vi "Model - Init.vi"(8 "error in (no error)":errorcluster) -> (0 "error out":errorcluster, 3 "View Model":T1)   [LabVIEW 2017]
doc: "Initializes View model's user events and DVRs"
uses:
  Controls/View Model.ctl
  Configuration/Controls/Config Model.ctl
  Configuration/Controls/Config Data.ctl
  Error Handler/Controls/Error Model.ctl
  Error Handler/Controls/Error Data.ctl
  Error Handler/Controls/Error Type.ctl
  Controls/Shared Model.ctl
  Elevator Controller/Controls/Elevator Model.ctl
  Elevator Controller/Controls/Elevator Location.ctl
  Elevator Controller/Controls/Elevator CMD Data.ctl
  Elevator Controller/Controls/Elevator Commands.ctl
  Elevator Controller/Controls/Elevator Overhead.ctl
  Elevator Controller/Controls/Elevator States.ctl
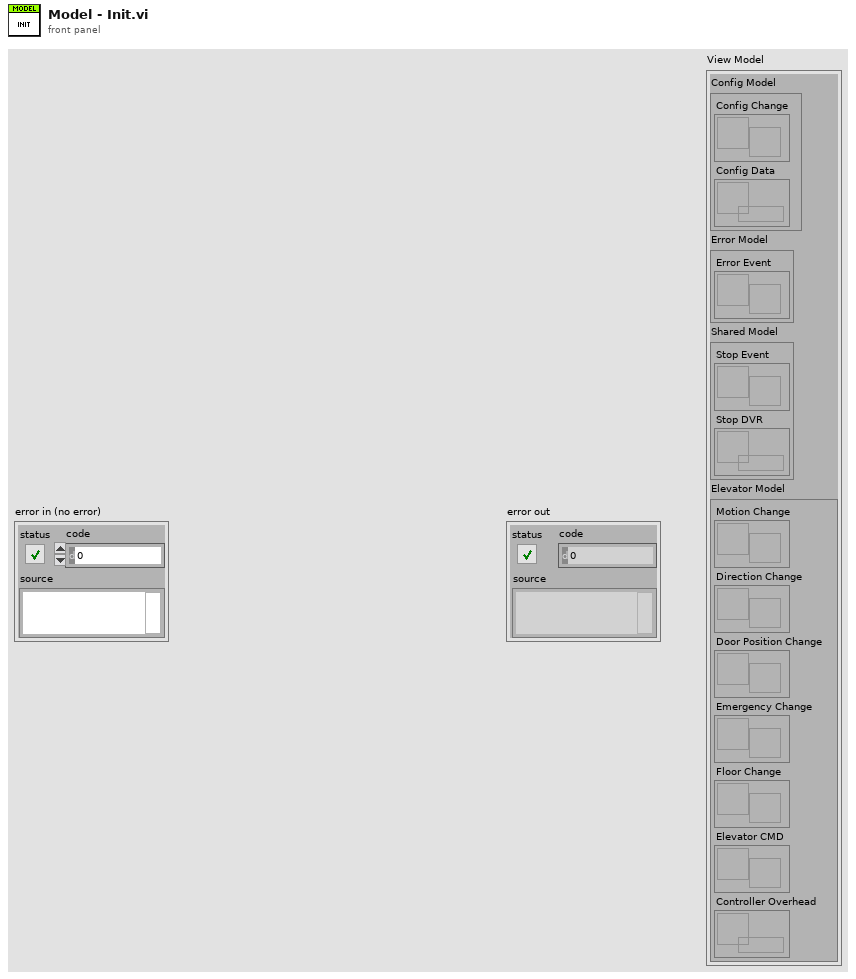
[diagram p1: front panel]
types:
  T1 = typedef "View Model.ctl" = cluster{"Config Model":T2, "Error Model":T3, "Shared Model":T4, "Elevator Model":T5}
  T2 = typedef "Config Model.ctl" = cluster{"Config Change":refnum<user-event>, "Config Data":refnum<data-value>}
  T3 = typedef "Error Model.ctl" = cluster{"Error Event":refnum<user-event>}
  T4 = typedef "Shared Model.ctl" = cluster{"Stop Event":refnum<user-event>, "Stop DVR":refnum<data-value>}
  T5 = typedef "Elevator Model.ctl" = cluster{"Motion Change":refnum<user-event>, "Direction Change":refnum<user-event>, "Door Position Change":refnum<user-event>, "Emergency Change":refnum<user-event>, "Floor Change":refnum<user-event>, "Elevator CMD":refnum<user-event>, "Controller Overhead":refnum<data-value>}
  T6 = typedef "Config Data.ctl" = cluster{"Door Open":dbl, "Door Close":dbl, "Travel Time":dbl, "Inactivity Time":dbl}
  T7 = typedef "Elevator CMD Data.ctl" = cluster{"Elevator Commands":T8, "Variant":variant}
  T8 = typedef "Elevator Commands.ctl" = enum16{"Go Up", "Go Down", "Go to Floor", "Emergency", "Open Doors", "Close Doors"}
  T9 = typedef "Elevator Location.ctl" = enum16{"1st Floor", "2nd Floor", "3rd Floor", "4th Floor"}
  T10 = typedef "Elevator Overhead.ctl" = cluster{"In Motion?":bool, "Direction":bool, "Door Movement":bool, "Timer":dbl, "Elapsed Time":dbl, "Door Position":bool, "Elevator State":T11, "Next Elevator State":T11}
  T11 = typedef "Elevator States.ctl" = enum16{"Idle", "Init", "Open Doors", "Close Doors", "Start Move", "Move", "Finish Move", "Emergency", "Analysis", "Terminate"}
  T12 = typedef "Error Data.ctl" = cluster{"Error Type":T13, "Variant":variant}
  T13 = typedef "Error Type.ctl" = enum16{"Console Error", "Process Step Error", "Sensor Interface IO Error"}
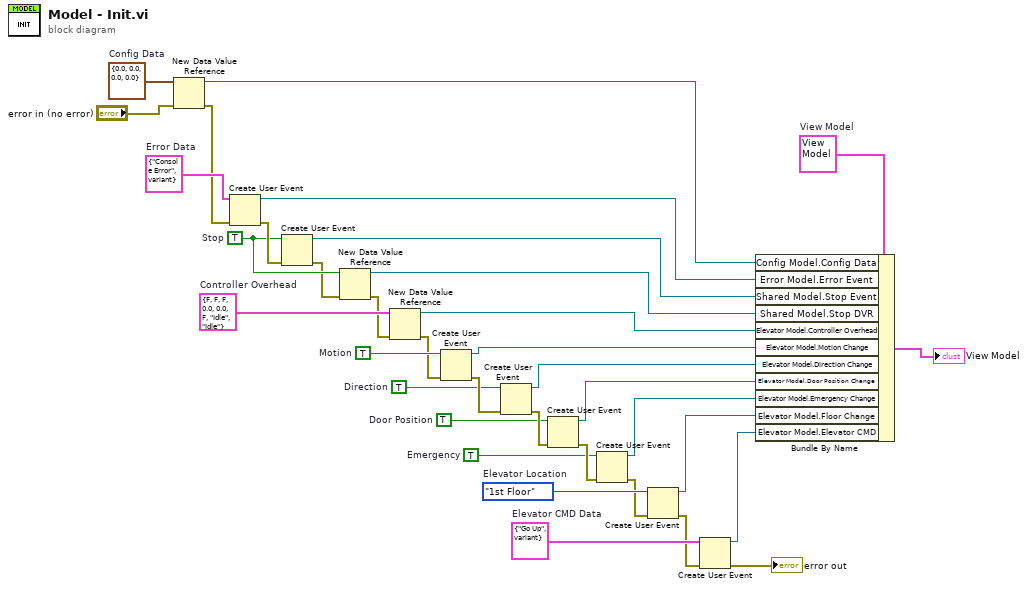
[diagram p0: block diagram]
diagram:
  w4 = T6 {"Door Open"=0.0, "Door Close"=0.0, "Travel Time"=0.0, "Inactivity Time"=0.0}  # Config Data
  w18 = T7 {"Elevator Commands"=enum."Go Up", "Variant"=variant}  # Elevator CMD Data
  w20 = Elevator_Location."1st Floor"  # Elevator Location
  w21 = TRUE  # Emergency
  w23 = TRUE  # Door Position
  w25 = TRUE  # Direction
  w28 = TRUE  # Motion
  w30 = T10 {"In Motion?"=FALSE, "Direction"=FALSE, "Door Movement"=FALSE, "Timer"=0.0, "Elapsed Time"=0.0, "Door Position"=FALSE, "Elevator State"=enum."Idle", "Next Elevator State"=enum."Idle"}  # Controller Overhead
  w32 = TRUE  # Stop
  w34 = T12 {"Error Type"=enum."Console Error", "Variant"=variant}  # Error Data
  w35 = T1 {"Config Model"={"Config Change"=refnum, "Config Data"=refnum}, "Error Model"={"Error Event"=refnum}, "Shared Model"={"Stop Event"=refnum, "Stop DVR"=refnum}, "Elevator Model"={"Motion Change"=refnum, "Direction Change"=refnum, "Door Position Change"=refnum, "Emergency Change"=refnum, "Floor Change"=refnum, "Elevator CMD"=refnum, "Controller Overhead"=refnum}}  # View Model
  n1 = New Data Value Reference(data value=w4, error in="error in (no error)") -> (data value reference=w1:refnum<data-value>, error out=w2:errorcluster)
  n2 = Create User Event(user event datatype=w34, error in=w2) -> (user event=w16:refnum<user-event>, error out=w33:errorcluster)
  n3 = Create User Event(user event datatype=w32, error in=w33) -> (user event=w15:refnum<user-event>, error out=w31:errorcluster)
  n4 = New Data Value Reference(data value=w32, error in=w31) -> (data value reference=w14:refnum<data-value>, error out=w29:errorcluster)
  n5 = New Data Value Reference(data value=w30, error in=w29) -> (data value reference=w13:refnum<data-value>, error out=w27:errorcluster)
  n6 = Create User Event(user event datatype=w28, error in=w27) -> (user event=w12:refnum<user-event>, error out=w26:errorcluster)
  n7 = Create User Event(user event datatype=w25, error in=w26) -> (user event=w11:refnum<user-event>, error out=w24:errorcluster)
  n8 = Create User Event(user event datatype=w23, error in=w24) -> (user event=w10:refnum<user-event>, error out=w22:errorcluster)
  n9 = Create User Event(user event datatype=w21, error in=w22) -> (user event=w9:refnum<user-event>, error out=w19:errorcluster)
  n10 = Create User Event(user event datatype=w20, error in=w19) -> (user event=w8:refnum<user-event>, error out=w17:errorcluster)
  n11 = Create User Event(user event datatype=w18, error in=w17) -> (user event=w7:refnum<user-event>, error out=→"error out":errorcluster)
  n12 = Bundle By Name(cluster=w35, "Config Model.Config Data"=w1, "Error Model.Error Event"=w16, "Shared Model.Stop Event"=w15, "Shared Model.Stop DVR"=w14, "Elevator Model.Controller Overhead"=w13, "Elevator Model.Motion Change"=w12, "Elevator Model.Direction Change"=w11, "Elevator Model.Door Position Change"=w10, "Elevator Model.Emergency Change"=w9, "Elevator Model.Floor Change"=w8, "Elevator Model.Elevator CMD"=w7) -> (→"View Model":T1)
